vi "Run Action.vi"(8 "error in (no error)":errorcluster, 10 "Action Data":T1, 11 "Project Action Interface in":refnum<class "Project Action Interface.lvclass">) -> (0 "error out":errorcluster, 1 "Success?":bool, 3 "Report Interface out":refnum<class "Report Data.lvclass">)   [LabVIEW 2020, in "ProjectBuilder.lvlib" / "Project Action Interface.lvclass"]
uses:
  Project Action Interface.lvclass
  Report Data/Report Data.lvclass
  Ctl/Ctl_Action Data.ctl
  ProjectBuilder.lvlib
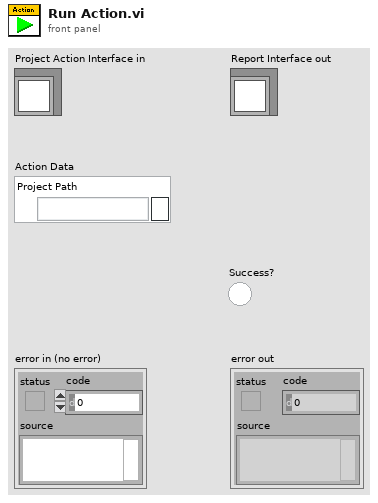
[diagram p1: front panel]
types:
  T1 = typedef "ProjectBuilder.lvlib/Ctl_Action Data.ctl" = cluster{"Project Path":path}
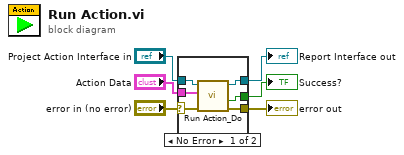
[diagram p0: block diagram]
diagram:
  n1 = case shown="No Error" "error in (no error)" {
    selector: "error in (no error)" -> [w12 w13]
    tunnel: [w11 w13] -> w5
    tunnel: [w9 _] -> w3
    tunnel: "Project Action Interface in" -> [w10 _]
    tunnel: [w8 _] -> w2
    tunnel: "Action Data" -> [w7 _]
    frame No Error {
      n2 = call-dynamic "Run Action_Do.vi"("error in (no error)"=w12, "Action Data"=w7, "Project Action Interface in"=w10) -> ("error out"=w11:errorcluster, "Success?"=w8:bool, "Report Interface out"=w9:refnum<class "Report Data.lvclass">)  [unwired: 6 in]
    }
    frame Error {
    }
  }
  "error out" <- w5
  "Report Interface out" <- w3
  "Success?" <- w2
